vi "Message Comparator.vi"(11 "Consumer Data Out in":T1 {"MIDI Parse Data"."Current Byte" format="%.0x"; "MIDI Parse Data"."Running Statusbyte" format="%.0x"; "MIDI Parse Data"."MIDI-Bytes In" format="%.0x"}) -> (3 "Consumer Data Out out":T1 {"MIDI Parse Data"."Current Byte" format="%.0x"; "MIDI Parse Data"."Running Statusbyte" format="%.0x"; "MIDI Parse Data"."MIDI-Bytes In" format="%.0x"})   [LabVIEW 2019]
uses:
  Controls/Consumer_Data.ctl
  Common/Controls/Application_Message.ctl
  Common/Controls/Application_State.ctl
  Controls/Consumer_States.ctl
  Controls/Transfer_Data.ctl
  MIDI/Controls/MIDI-Message_Array.ctl
  MIDI/Controls/MIDI-Message_Cluster.ctl
  MIDI/Controls/Meta_Commands.ctl
  Controls/Parser-data.ctl
  Controls/Consumer_Result.ctl
  Controls/Parsed_Data.ctl
panel:
  out "String 2":string
  out "String":string
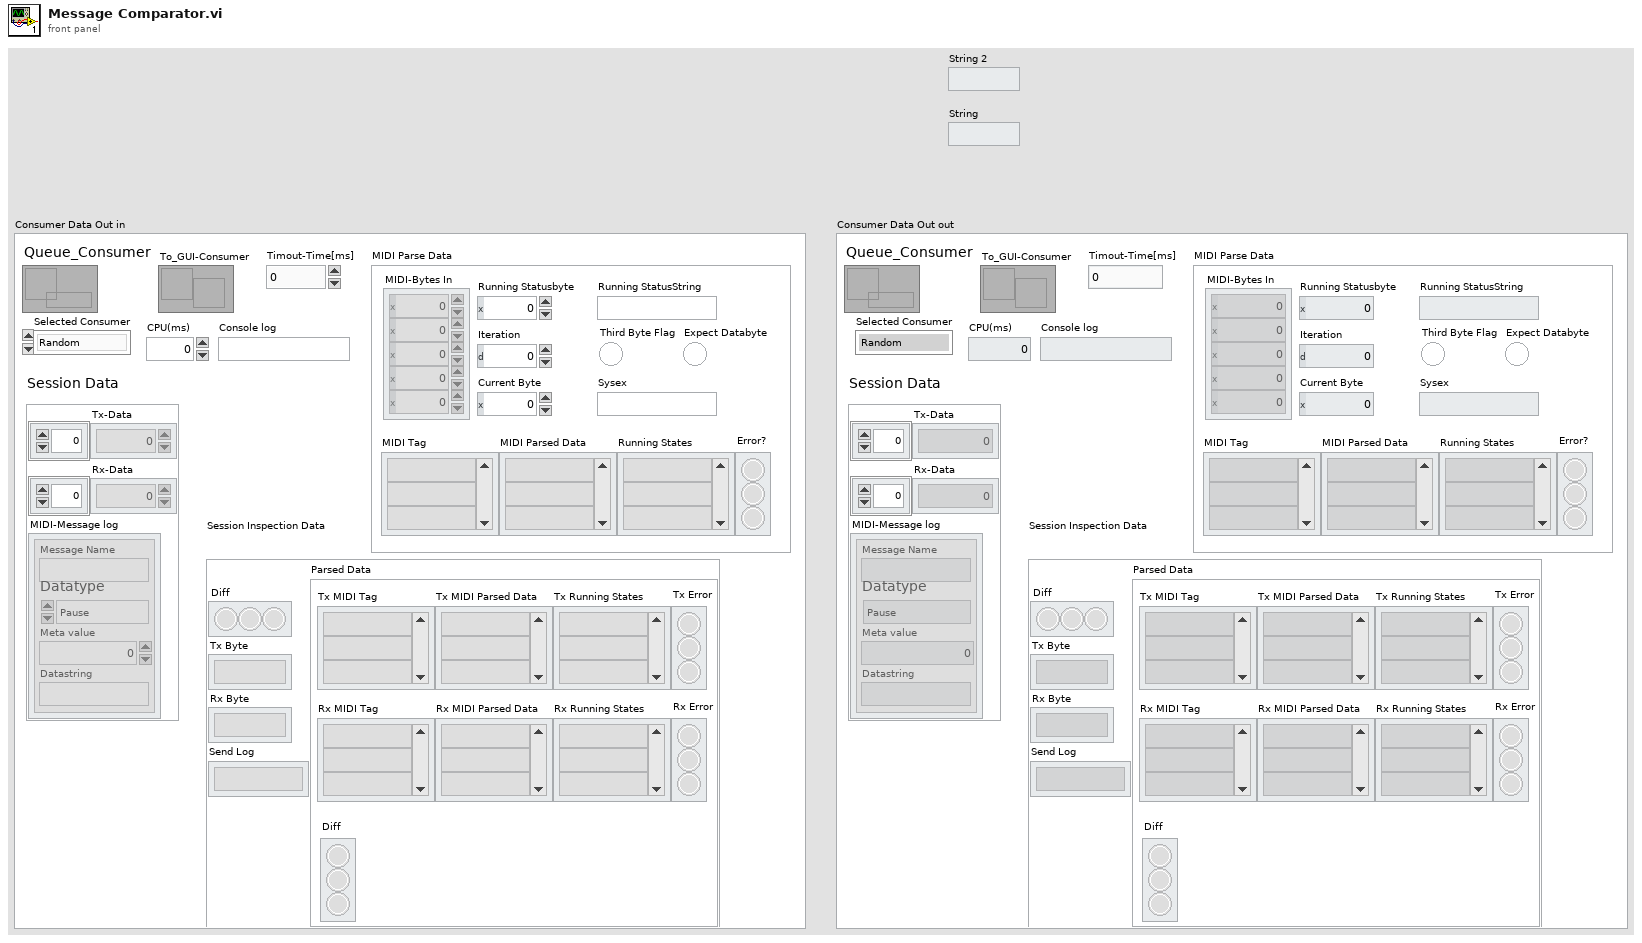
[diagram p1: front panel]
types:
  T1 = typedef "Consumer_Data.ctl" = cluster{"Queue_Consumer":refnum<queue>, "Selected Consumer":T2, "Session Data":T3, "Timout-Time[ms]":i32, "To_GUI-Consumer":refnum<user-event>, "CPU(ms)":u32, "Console log":string, "MIDI Parse Data":T7, "Session Inspection Data":T8}
  T2 = typedef "Consumer_States.ctl" = enum16{"Random", "ECG", "Strech-Patch"}
  T3 = typedef "Transfer_Data.ctl" = cluster{"Tx-Data":i8[], "Rx-Data":i8[], "MIDI-Message log":T4}
  T4 = typedef "MIDI-Message_Array.ctl" = T5[]
  T5 = typedef "MIDI-Message_Cluster.ctl" = cluster{"Message Name":string, "Meta value":i32, "Datastring":string, "Datatype":T6}
  T6 = typedef "Meta_Commands.ctl" = enum16{"No Data", "Pause", "Loop", "Wait for Rx", "Delay", "Break", "MIDI"}
  T7 = typedef "Parser-data.ctl" = cluster{"MIDI-Bytes In":u8[], "MIDI Tag":string[], "MIDI Parsed Data":string[], "Iteration":i32, "Error?":bool[], "Running States":string[], "Running Statusbyte":u8, "Running StatusString":string, "Third Byte Flag":bool, "Current Byte":u8, "Sysex":string, "Expect Databyte":bool}
  T8 = typedef "Consumer_Result.ctl" = cluster{"Diff":bool[], "Tx Byte":string[], "Rx Byte":string[], "Send Log":string[], "Parsed Data":T9}
  T9 = typedef "Parsed_Data.ctl" = cluster{"Tx MIDI Tag":string[], "Tx MIDI Parsed Data":string[], "Tx Error":bool[], "Tx Running States":string[], "Rx MIDI Tag":string[], "Rx MIDI Parsed Data":string[], "Rx Error":bool[], "Rx Running States":string[], "Diff":bool[]}
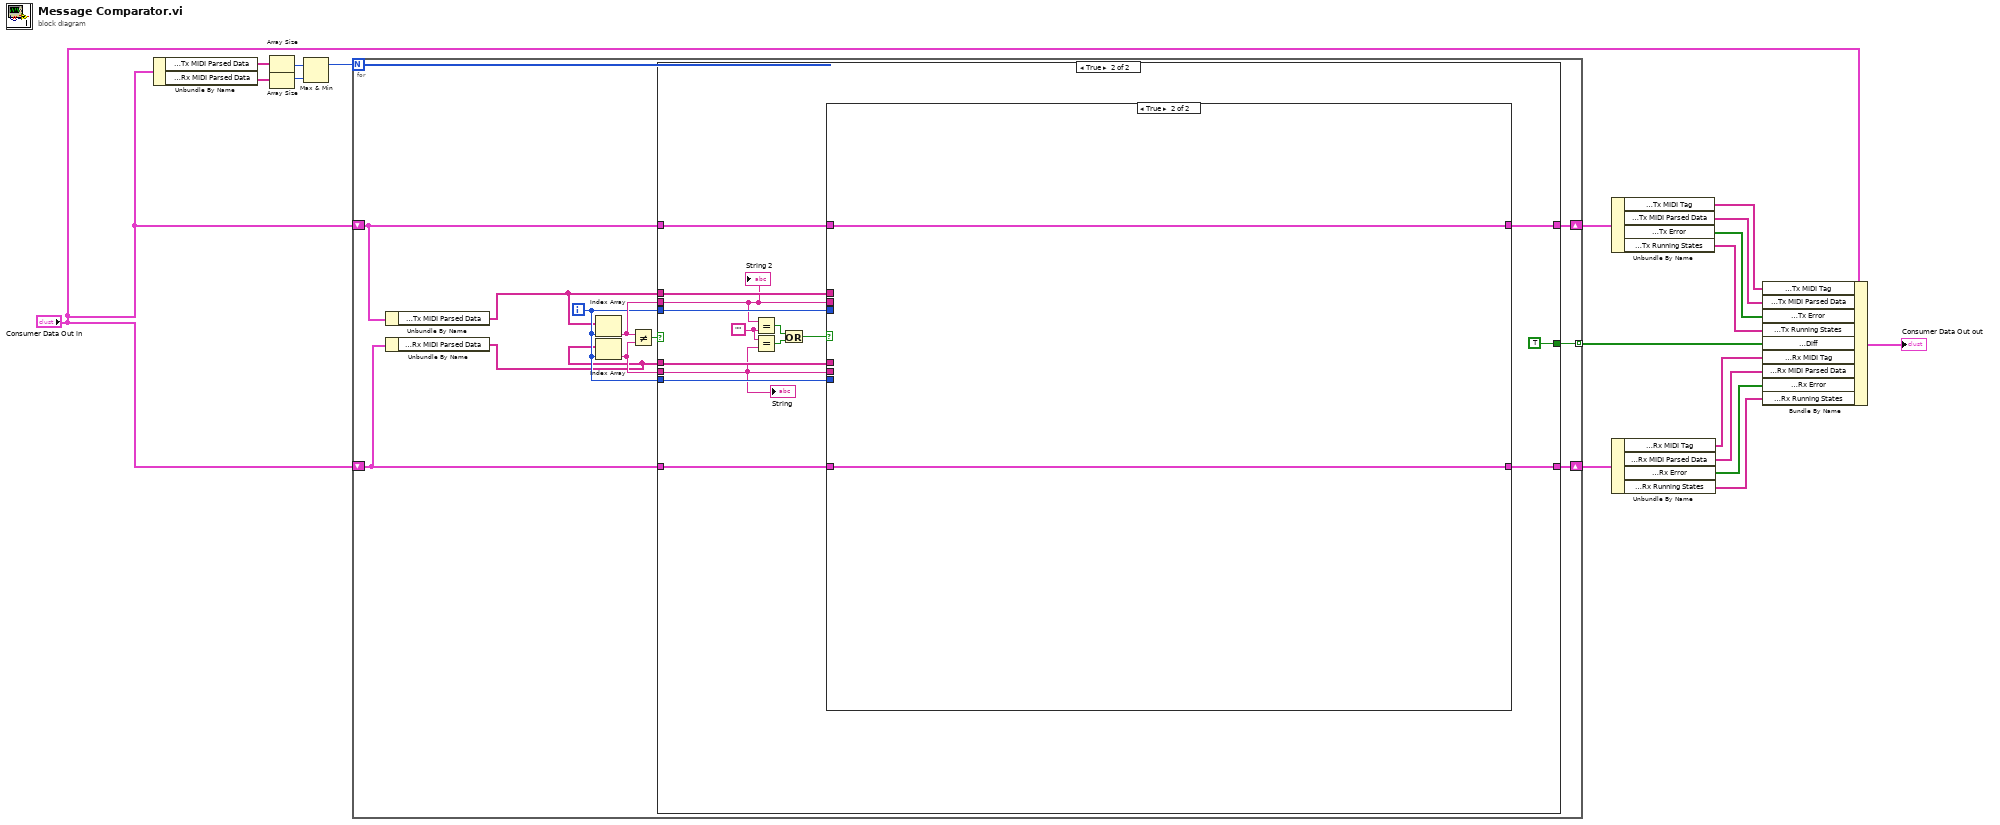
[diagram p0: block diagram]
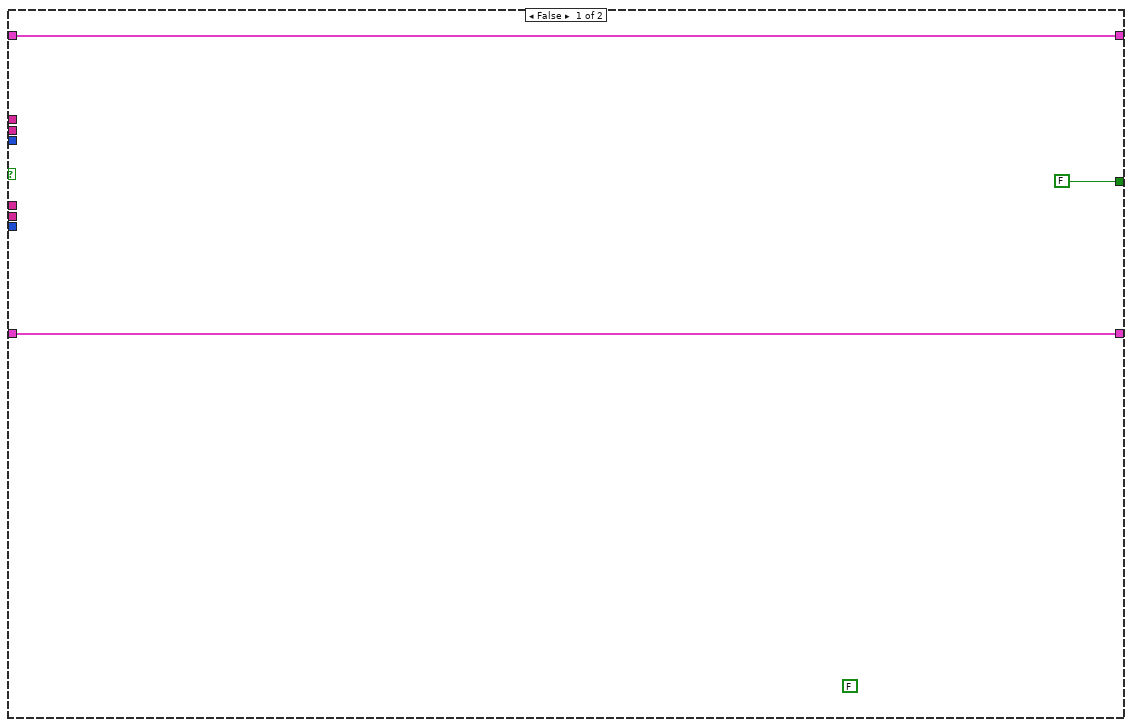
[diagram p2: hidden frame]
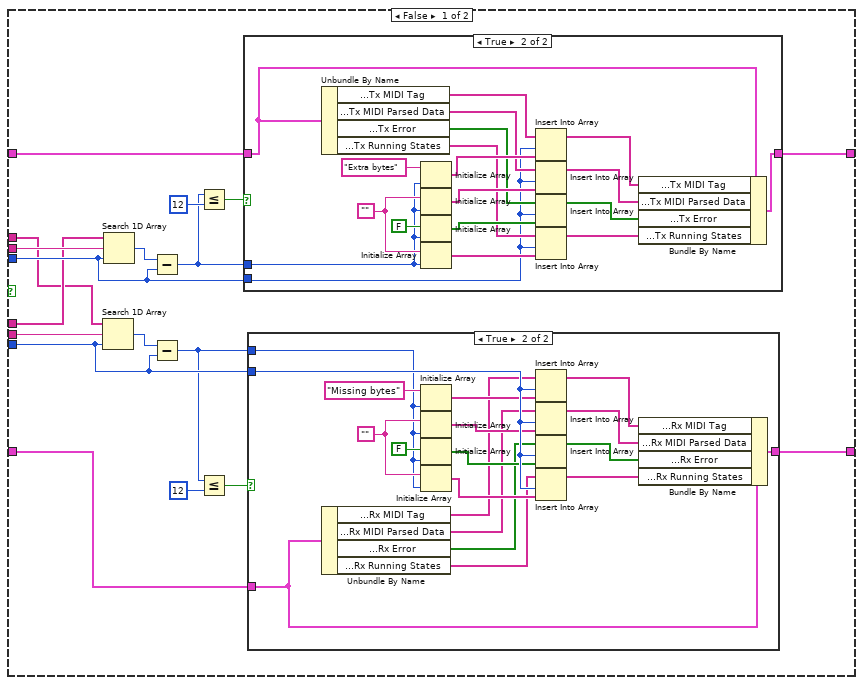
[diagram p3: hidden frame]
diagram:
  n1 = Unbundle By Name("Consumer Data Out in") -> ("Session Inspection Data.Parsed Data.Tx MIDI Parsed Data"=w17:string[], "Session Inspection Data.Parsed Data.Rx MIDI Parsed Data"=w18:string[])
  n2 = Array Size(array=w17) -> (size(s)=w15:i32)
  n3 = Array Size(array=w18) -> (size(s)=w14:i32)
  n4 = Max & Min(x=w15, y=w14) -> (max(x,y)=w16:i32)  [unwired: 1 out]
  n5 = for {
    N: w16 -> [_]
    tunnel: [w25] -> w2 mode=indexing
    shift-right: [w24] -> w12
    shift-left: "Consumer Data Out in" -> [w21]
    shift-right: [w23] -> w7
    shift-left: "Consumer Data Out in" -> [w20]
    i -> [w26]
    n6 = Unbundle By Name(w21) -> ("Session Inspection Data.Parsed Data.Tx MIDI Parsed Data"=w22:string[])
    n7 = Unbundle By Name(w20) -> ("Session Inspection Data.Parsed Data.Rx MIDI Parsed Data"=w19:string[])
    n8 = Index Array(array=w22, index=w26) -> (element=w28:string)
    n9 = Index Array(array=w19, index=w26) -> (element=w27:string)
    n10 = Not Equal?(x=w28, y=w27) -> (x != y?=w29:bool)
    n11 = case shown="True" w29 {
      tunnel: w22 -> [_ w40]
      tunnel: w19 -> [_ w41]
      tunnel: w28 -> [_ w34]
      tunnel: w27 -> [_ w35]
      tunnel: w26 -> [_ w47]
      tunnel: w26 -> [_ w45]
      tunnel: w20 -> [w31 w44]
      tunnel: w21 -> [w32 w46]
      tunnel: [FALSE TRUE] -> w25
      tunnel: [w32 w43] -> w24
      tunnel: [w31 w42] -> w23
      frame False {
        (unwired) FALSE
      }
      frame True {
        w33 = "" ("y")
        n12 = Equal?(x=w34, y=w33) -> (x = y?=w37:bool)
        n13 = Equal?(x=w33, y=w35) -> (x = y?=w36:bool)
        n14 = Or(x=w37, y=w36) -> (x .or. y?=w38:bool)
        n15 = case shown="True" w38 {
          tunnel: w34 -> [w65 _]
          tunnel: w35 -> [w64 _]
          tunnel: w47 -> [w61 _]
          tunnel: w46 -> [w60 w106]
          tunnel: w45 -> [w59 _]
          tunnel: w44 -> [w58 w107]
          tunnel: [w52 w106] -> w43
          tunnel: [w51 w107] -> w42
          tunnel: w41 -> [w49 _]
          tunnel: w40 -> [w48 _]
          frame False {
            n16 = Search 1D Array(1D array=w48, element=w64, start index (0)=w59) -> (index of element=w62:i32)
            n17 = Search 1D Array(1D array=w49, element=w65, start index (0)=w61) -> (index of element=w63:i32)
            n18 = Subtract(x=w63, y=w61) -> (x-y=w53:i32)
            n19 = Subtract(x=w62, y=w59) -> (x-y=w57:i32)
            n20 = Less Or Equal?(x=w53, y=12) -> (x <= y?=w54:bool)
            n21 = Less Or Equal?(x=w57, y=12) -> (x <= y?=w50:bool)
            n22 = case shown="True" w54 {
              tunnel: w61 -> [_ w89]
              tunnel: w60 -> [w86 w94]
              tunnel: w53 -> [_ w87]
              tunnel: [w86 w88] -> w52
              frame False {
              }
              frame True {
                w96 = ""
                n23 = Unbundle By Name(w94) -> ("Session Inspection Data.Parsed Data.Tx MIDI Tag"=w101:string[], "Session Inspection Data.Parsed Data.Tx MIDI Parsed Data"=w100:string[], "Session Inspection Data.Parsed Data.Tx Error"=w99:bool[], "Session Inspection Data.Parsed Data.Tx Running States"=w98:string[])
                n24 = Initialize Array("Extra bytes", w87) -> (w102:string[])
                n25 = Initialize Array(w96, w87) -> (w103:string[])
                n26 = Initialize Array(FALSE, w87) -> (w104:bool[])
                n27 = Initialize Array(w96, w87) -> (w105:string[])
                n28 = Insert Into Array(array=w101, index=w89, new element=w102) -> (w93:string[])
                n29 = Insert Into Array(array=w100, index=w89, new element=w103) -> (w92:string[])
                n30 = Insert Into Array(array=w99, index=w89, new element=w104) -> (w91:bool[])
                n31 = Insert Into Array(array=w98, index=w89, new element=w105) -> (w90:string[])
                n32 = Bundle By Name(cluster=w94, "Session Inspection Data.Parsed Data.Tx MIDI Tag"=w93, "Session Inspection Data.Parsed Data.Tx MIDI Parsed Data"=w92, "Session Inspection Data.Parsed Data.Tx Error"=w91, "Session Inspection Data.Parsed Data.Tx Running States"=w90) -> (w88:T1)
              }
            }
            n33 = case shown="True" w50 {
              tunnel: w59 -> [_ w82]
              tunnel: w58 -> [w66 w67]
              tunnel: w57 -> [_ w69]
              tunnel: [w66 w68] -> w51
              frame False {
              }
              frame True {
                w84 = ""
                n34 = Unbundle By Name(w67) -> ("Session Inspection Data.Parsed Data.Rx MIDI Tag"=w77:string[], "Session Inspection Data.Parsed Data.Rx MIDI Parsed Data"=w76:string[], "Session Inspection Data.Parsed Data.Rx Error"=w75:bool[], "Session Inspection Data.Parsed Data.Rx Running States"=w74:string[])
                n35 = Initialize Array("Missing bytes", w69) -> (w81:string[])
                n36 = Initialize Array(w84, w69) -> (w80:string[])
                n37 = Initialize Array(FALSE, w69) -> (w79:bool[])
                n38 = Initialize Array(w84, w69) -> (w78:string[])
                n39 = Insert Into Array(array=w77, index=w82, new element=w81) -> (w73:string[])
                n40 = Insert Into Array(array=w76, index=w82, new element=w80) -> (w72:string[])
                n41 = Insert Into Array(array=w75, index=w82, new element=w79) -> (w71:bool[])
                n42 = Insert Into Array(array=w74, index=w82, new element=w78) -> (w70:string[])
                n43 = Bundle By Name(cluster=w67, "Session Inspection Data.Parsed Data.Rx MIDI Tag"=w73, "Session Inspection Data.Parsed Data.Rx MIDI Parsed Data"=w72, "Session Inspection Data.Parsed Data.Rx Error"=w71, "Session Inspection Data.Parsed Data.Rx Running States"=w70) -> (w68:T1)
              }
            }
          }
          frame True {
          }
        }
        "String" <- w35
        "String 2" <- w34
      }
    }
  }
  n44 = Unbundle By Name(w12) -> ("Session Inspection Data.Parsed Data.Tx MIDI Tag"=w11:string[], "Session Inspection Data.Parsed Data.Tx MIDI Parsed Data"=w10:string[], "Session Inspection Data.Parsed Data.Tx Error"=w9:bool[], "Session Inspection Data.Parsed Data.Tx Running States"=w8:string[])
  n45 = Unbundle By Name(w7) -> ("Session Inspection Data.Parsed Data.Rx MIDI Tag"=w6:string[], "Session Inspection Data.Parsed Data.Rx MIDI Parsed Data"=w5:string[], "Session Inspection Data.Parsed Data.Rx Error"=w4:bool[], "Session Inspection Data.Parsed Data.Rx Running States"=w3:string[])
  n46 = Bundle By Name(cluster="Consumer Data Out in", "Session Inspection Data.Parsed Data.Tx MIDI Tag"=w11, "Session Inspection Data.Parsed Data.Tx MIDI Parsed Data"=w10, "Session Inspection Data.Parsed Data.Tx Error"=w9, "Session Inspection Data.Parsed Data.Tx Running States"=w8, "Session Inspection Data.Parsed Data.Diff"=w2, "Session Inspection Data.Parsed Data.Rx MIDI Tag"=w6, "Session Inspection Data.Parsed Data.Rx MIDI Parsed Data"=w5, "Session Inspection Data.Parsed Data.Rx Error"=w4, "Session Inspection Data.Parsed Data.Rx Running States"=w3) -> (→"Consumer Data Out out":T1)
